vi "delays_insert.vi"(0 "From full":bool=TRUE, 3 "Delays / fs":dbl[](array[numeric])=[-500.0, -250.0, -100.0, -50.0, -25.0, 0.0, 25.0, 50.0, 100.0, 250.0, 1000.0, 3000.0, 5000.0], 4 "Delays in":string[][](array[string]), 5 "t0 / mm":dbl) -> (2 "Delays_out":string[][](array[string]))   [LabVIEW 2019]
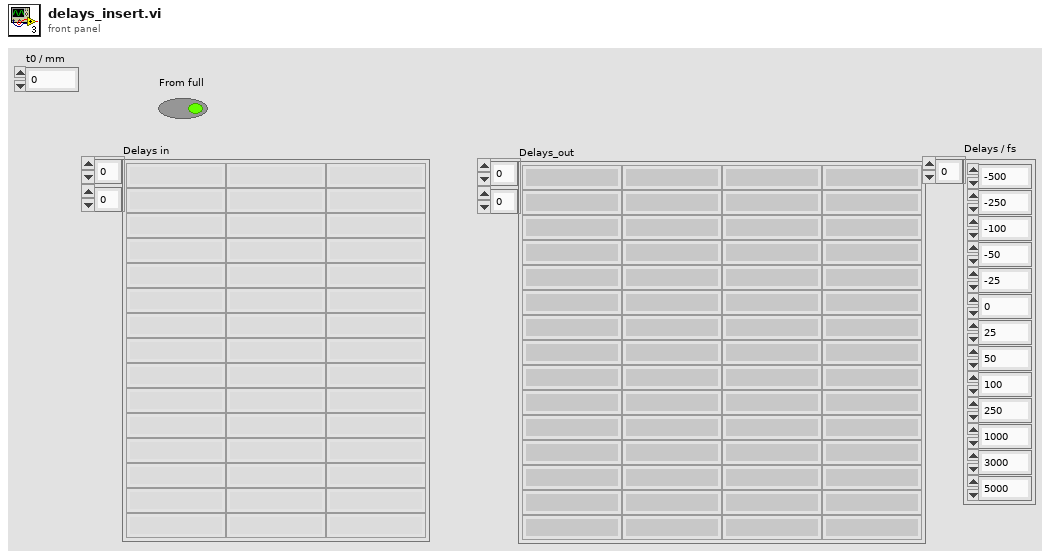
[diagram p1: front panel]
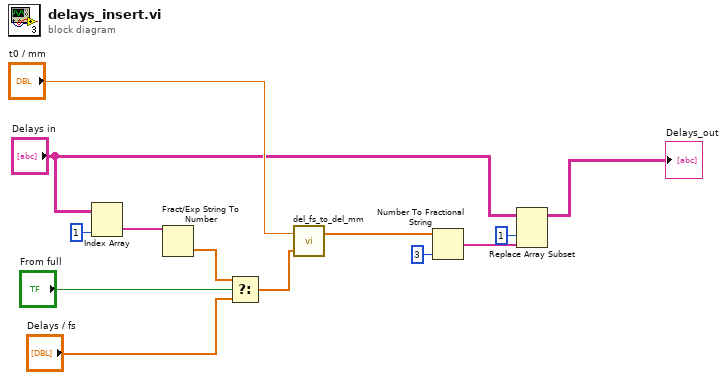
[diagram p0: block diagram]
diagram:
  n1 = Index Array(array="Delays in", index (col)=1 ("disabled index (col)")) -> (element=w12:string[])  [unwired: 1 in]
  n2 = Fract/Exp String To Number(string=w12) -> (number=w3:dbl[])  [unwired: 3 in, 1 out]
  n3 = Select(t=w3, s="From full", f="Delays / fs") -> (s? t:f=w1:dbl[])
  n4 = call "del_fs_to_del_mm.vi"("Delays / fs"=w1, "t0 / mm"="t0 / mm") -> ("Delays / mm"=w10:dbl[])  [unwired: 1 in]
  n5 = Number To Fractional String(number=w10, precision (6)=i16 3) -> (F-format string=w7:string[])  [unwired: 2 in]
  n6 = Replace Array Subset(array="Delays in", new element=w7, index (col)=1 ("disabled index (col)")) -> (→"Delays_out":string[][])  [unwired: 1 in]
